vi "Log RT Driver Error.vi"(8 "error in":errorcluster) -> ()   [LabVIEW 2020, in "AIM MIL-STD-1553 Engine.lvlib" / "Custom Device.lvlib"]
uses:
  Custom Device.lvlib
  <vilib>/NI VeriStand/Custom Device Tools/Custom Device Utility Library/Custom Device Utility Library.lvlib
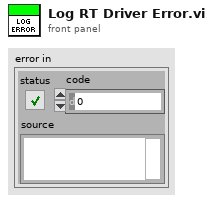
[diagram p1: front panel]
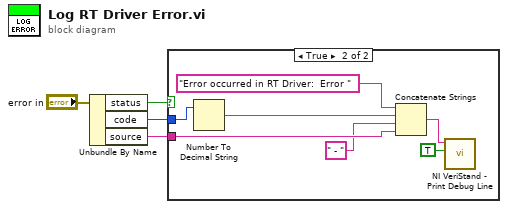
[diagram p0: block diagram]
diagram:
  n1 = Unbundle By Name("error in") -> ("status"=w3:bool, "code"=w1:i32, "source"=w2:string)
  n2 = case shown="True" w3 {
    tunnel: w2 -> [_ w7]
    tunnel: w1 -> [_ w8]
    frame False {
    }
    frame True {
      n3 = Number To Decimal String(number=w8) -> (decimal integer string=w10:string)  [unwired: 1 in]
      n4 = Concatenate Strings("Error occurred in RT Driver:  Error ", w10, " - ", w7) -> (w9:string)
      n5 = call <vilib>:"NI VeriStand - Print Debug Line.vi"("Add to log file? (F)"=TRUE, "Message"=w9) -> ()  [unwired: 9 in, 1 out]
    }
  }
